vi "пр1_2.vi"() -> ()   [LabVIEW 2010]
panel:
  in  "E":dbl(slide) scale=0.0..10.0
  out "I 3":dbl(knob) scale=0.0..10.0
  out "I 2":dbl(knob) scale=0.0..10.0
  out "I1":dbl(knob) scale=0.0..10.0
  in  "R3":dbl(knob) scale=0.0..10.0
  in  "R2":dbl(knob) scale=0.0..10.0
  in  "R1":dbl(knob) scale=0.0..10.0
  # "I1"
  # "R1"
  # "I2"
  # "I3"
  # "E"
  # "R2"
  # "R3"
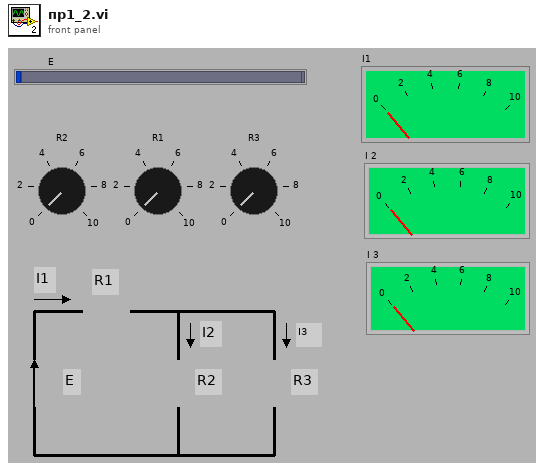
[diagram p1: front panel]
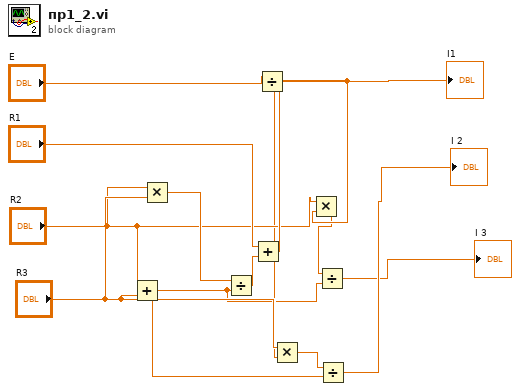
[diagram p0: block diagram]
diagram:
  n1 = Add(x="R2", y="R3") -> (x+y=w2:dbl)
  n2 = Multiply(x="R2", y="R3") -> (x*y=w13:dbl)
  n3 = Divide(x=w13, y=w2) -> (x/y=w11:dbl)
  n4 = Add(x="R1", y=w11) -> (x+y=w10:dbl)
  n5 = Divide(x="E", y=w10) -> (x/y=w4:dbl)
  "I1" <- w4
  n6 = Multiply(x="R3", y=w4) -> (x*y=w7:dbl)
  n7 = Multiply(x="R2", y=w4) -> (x*y=w3:dbl)
  n8 = Divide(x=w3, y=w2) -> (x/y=→"I 3":dbl)
  n9 = Divide(x=w7, y=w2) -> (x/y=→"I 2":dbl)
